vi "CRYRead Harmonics list file.vi"(11 "String":string) -> (3 "Harmonics list":string[](array[string]))   [LabVIEW 2013]
uses:
  CRYMainGlobal.vi
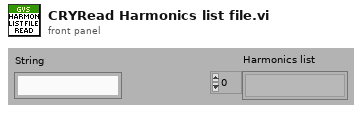
[diagram p1: front panel]
types:
  T1 = enum16{"read/write", "read-only", "write-only", "write-only (truncate)"}
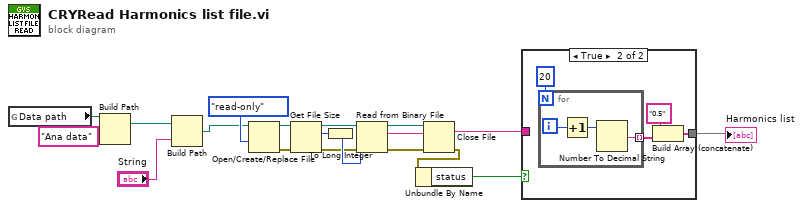
[diagram p0: block diagram]
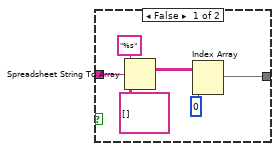
[diagram p2: hidden frame]
diagram:
  n1 = global read "CRYMainGlobal.vi" "Data path"() -> (w1:path)
  n2 = Build Path(base path=w1, name or relative path="Ana data") -> (appended path=w7:path)
  n3 = Build Path(base path=w7, name or relative path="String") -> (appended path=w2:path)
  n4 = Open/Create/Replace File(file path (use dialog)=w2, access (0:read/write)=T1."read-only" ("open mode (0)")) -> (refnum out=w8:refnum<file>, error out=w16:errorcluster)  [unwired: 1 in, 4 out]
  n5 = Get File Size(file=w8, error in=w16) -> (refnum out=w13:refnum<file>, size (in bytes)=w9:i64, 0:w14:errorcluster)
  n6 = To Long Integer(number=w9) -> (32bit integer=w15:i32)
  n7 = Read from Binary File(8:w14, 10:w15, 11:w13) -> (0:w11:errorcluster, 2:w6:string, 3:w12:refnum<file>)  [unwired: 4 out]
  n8 = Close File(refnum=w12, error in=w11) -> (error out=w10:errorcluster)  [unwired: 1 out]
  n9 = Unbundle By Name(w10) -> ("status"=w5:bool)
  n10 = case shown="True" w5 {
    tunnel: w6 -> [w22 _]
    tunnel: [w19 w25] -> w4
    frame False {
      n11 = Spreadsheet String To Array(format string="%s", spreadsheet string=w22, array type (2D Dbl)=string[][] []) -> (array=w20:string[][])  [unwired: 1 out]
      n12 = Index Array(array=w20, index (col)=0 ("Index")) -> (element=w19:string[])  [unwired: 1 in]
    }
    frame True {
      n13 = for {
        N: 20 -> [_]
        tunnel: [w29] -> w28 mode=indexing
        i -> [w31]
        n14 = Increment(x=w31) -> (x+1=w30:i32)
        n15 = Number To Decimal String(number=w30) -> (decimal integer string=w29:string)  [unwired: 1 out]
      }
      n16 = Build Array (concatenate)("0.5", w28) -> (w25:string[])
    }
  }
  "Harmonics list" <- w4
